vi "NiFPGA Acknowledge IRQs.vi"(8 "error in (no error)":errorcluster, 10 "IRQs":u32, 11 "Session In":u32) -> (0 "error out":errorcluster, 3 "Session Out":u32)   [LabVIEW 2010, in "FPGA Interface Wrapper.lvlib"]
doc: "Acknowledges an IRQ or set of IRQs."
uses:
  <userlib>/_FPGA Interface Advanced Tools/FPGA Interface Wrapper/FPGA Interface Wrapper.lvlib
  NiFpga.dll
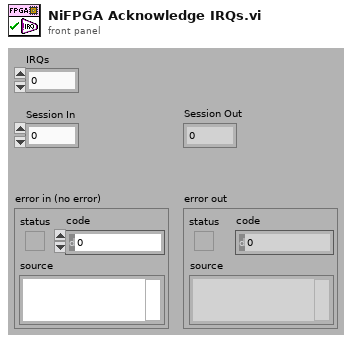
[diagram p1: front panel]
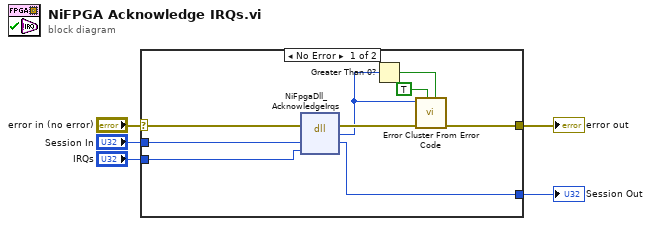
[diagram p0: block diagram]
diagram:
  n1 = case shown="No Error" "error in (no error)" {
    selector: "error in (no error)" -> [w14 w15]
    tunnel: [w6 w15] -> w5
    tunnel: [w13 w16] -> w3
    tunnel: "Session In" -> [w12 w16]
    tunnel: "IRQs" -> [w11 _]
    frame No Error {
      n2 = dll-call lib="NiFpga.dll" fn="NiFpgaDll_AcknowledgeIrqs"(error in=w14, "Session"=w12, "IRQs"=w11) -> (error out=w8:errorcluster, "Status"=w7:i32, "Session"=w13:u32)  [unwired: 3 in, 1 out]
      n3 = Greater Than 0?(x=w7) -> (x > 0?=w9:bool)
      n4 = call <vilib>:"Error Cluster From Error Code.vi"("is warning? (False)"=w9, "show call chain? (False)"=TRUE, "error in (no error)"=w8, "error code (0)"=w7) -> ("error out"=w6:errorcluster)  [unwired: 5 in]
    }
    frame Error {
    }
  }
  "error out" <- w5
  "Session Out" <- w3
